vi "forcesim.vi"(2 "Phase":dbl, 3 "dT":dbl, 4 "Speed":dbl) -> (0 "Force":dbl, 1 "Phase Out":dbl)   [LabVIEW 2025]
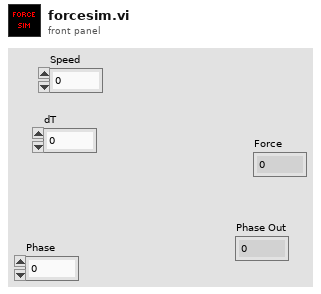
[diagram p1: front panel]
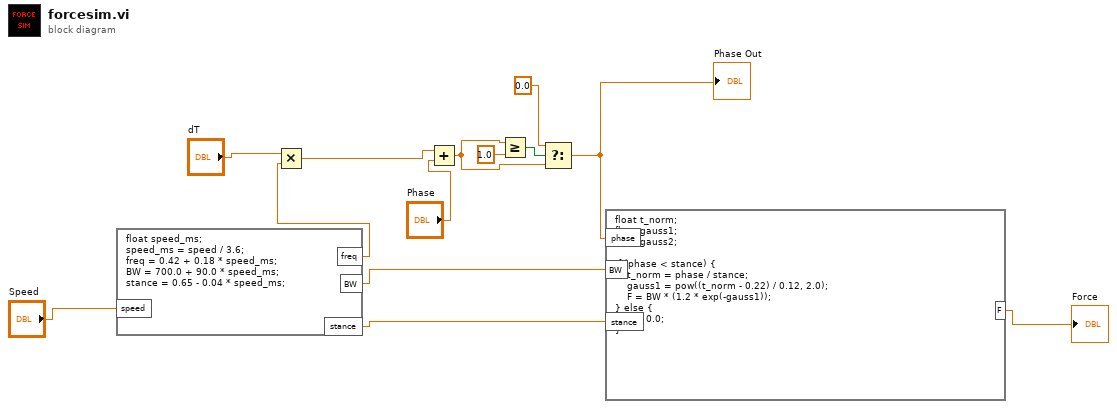
[diagram p0: block diagram]
diagram:
  n1 = formula code="float speed_ms;\nspeed_ms = speed / 3.6;\nfreq = 0.42 + 0.18 * speed_ms;\nBW = 700.0 + 90.0 * speed_ms;\nstance = 0.65 - 0.04 * speed_ms;"("speed"="Speed") -> ("freq"=w11:dbl, "BW"=w3:dbl, "stance"=w4:dbl)
  n2 = Multiply(x="dT", y=w11) -> (x*y=w10:dbl)
  n3 = Add(x=w10, y="Phase") -> (x+y=w5:dbl)
  n4 = Greater Or Equal?(x=w5, y=1.0) -> (x >= y?=w7:bool)
  n5 = Select(t=0.0 ("y"), s=w7, f=w5) -> (s? t:f=w1:dbl)
  "Phase Out" <- w1
  n6 = formula code="float t_norm;\nfloat gauss1;\nfloat gauss2;\n\nif (phase < stance) {\n    t_norm = phase / stance;\n    gauss1 = pow((t_norm - 0.22) / 0.12, 2.0);\n    F = BW * (1.2 * exp(-gauss1));\n} else {\n    F = 0.0;\n}"("phase"=w1, "BW"=w3, "stance"=w4) -> ("F"=→"Force":dbl)
